vi "wave-output.vi"() -> ()   [LabVIEW 2013]
panel:
  in  "Volt-Lbs Intercept":dbl
  in  "Volts-Lbs coeff.":dbl
  out "Volts-Lbs":dynamicdata(graph)
  out "Raw Volts":dynamicdata(graph)
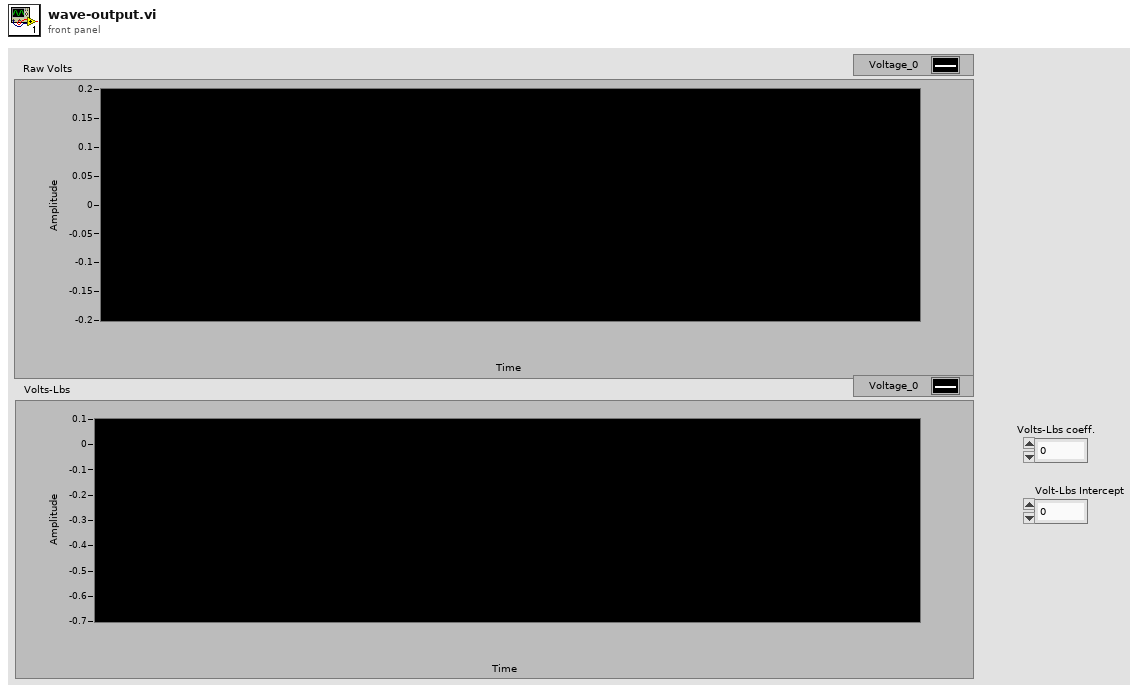
[diagram p1: front panel]
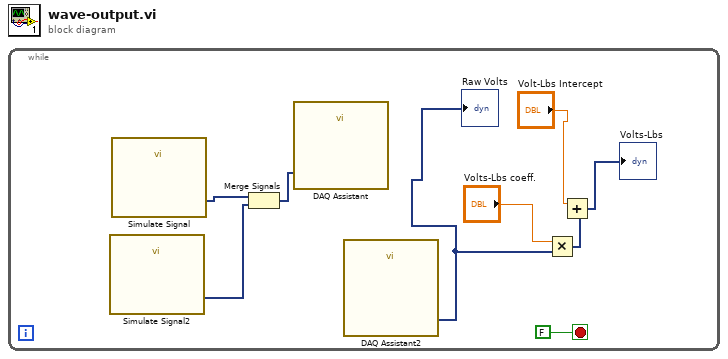
[diagram p0: block diagram]
diagram:
  n1 = while {
    stop <- FALSE stop-if-true
    n2 = call "Simulate Signal2"() -> ("DC"=w7:dynamicdata)  [unwired: 14 in, 1 out]
    n3 = call "Simulate Signal"() -> ("DC"=w9:dynamicdata)  [unwired: 14 in, 1 out]
    n4 = Merge Signals(w9, w7) -> (w8:dynamicdata)
    n5 = call "DAQ Assistant"("data"=w8) -> ()  [unwired: 16 in, 3 out]
    n6 = call "DAQ Assistant2"() -> ("data"=w6:dynamicdata)  [unwired: 16 in, 3 out]
    "Raw Volts" <- w6
    n7 = Multiply(x="Volts-Lbs coeff.", y=w6) -> (x*y=w3:dynamicdata)
    n8 = Add(x="Volt-Lbs Intercept", y=w3) -> (x+y=→"Volts-Lbs":dynamicdata)
  }
